vi "Stable.vi"(8 "Eval Period (sec)":dbl(knob)=0.5044674819294696 scale=0.0..1.0, 11 "Signal Input":bool) -> (0 "Stable":bool)   [LabVIEW 2011]
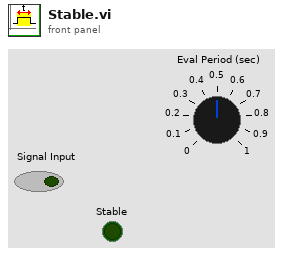
[diagram p1: front panel]
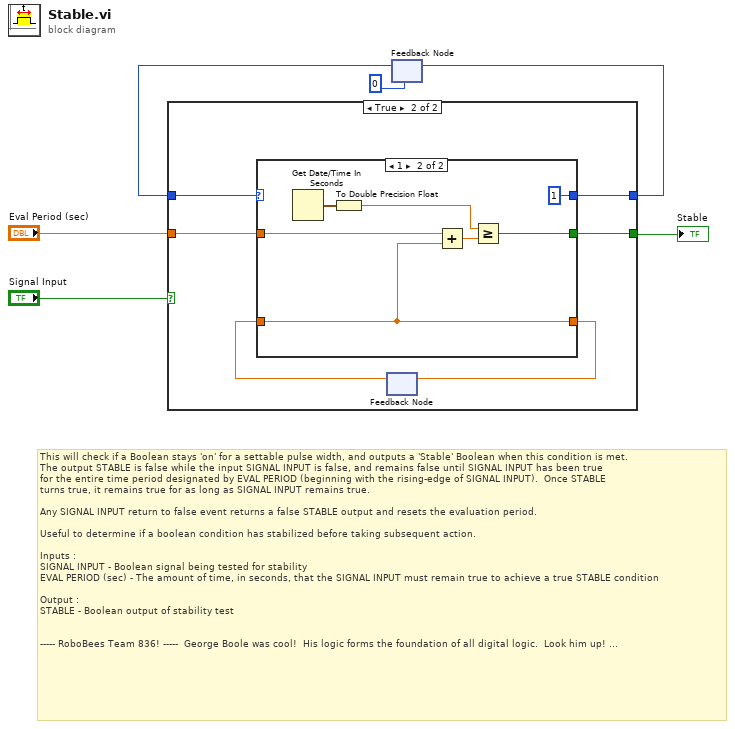
[diagram p0: block diagram]
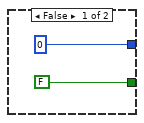
[diagram p2: hidden frame]
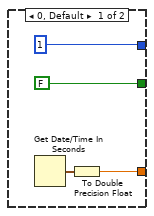
[diagram p3: hidden frame]
diagram:
  # "This will check if a Boolean stays 'on' for a settable pulse width, and outputs a 'Stable' Boolean when this condition is met.\nThe output STABLE is false while the input SIGNAL INPUT is false, and remains false until SIGNAL INPUT has been true\nfor the entire time period designated by EVAL PERIOD (beginning with the rising-edge of SIGNAL INPUT).  Once STABLE \nturns true, it remains true for as long as SIGNAL INPUT remains true.\n\nAny SIGNAL INPUT return to false event returns a false STABLE output and resets the evaluation period.\n\nUseful to determine if a boolean condition has stabilized before taking subsequent action.\n\nInputs :\nSIGNAL INPUT - Boolean signal being tested for stability\nEVAL PERIOD (sec) - The amount of time, in seconds, that the SIGNAL INPUT must remain true to achieve a true STABLE condition\n\nOutput :\nSTABLE - Boolean output of stability test\n\n\n----- RoboBees Team 836! -----  George Boole was cool!  His logic forms the foundation of all digital logic.  Look him up! ..."
  n1 = feedback #1(0) -> (w1:i32)
  n2 = case shown="True" "Signal Input" {
    tunnel: [FALSE w14] -> w6
    tunnel: "Eval Period (sec)" -> [_ w13]
    tunnel: [0 w10] -> w2
    tunnel: w1 -> [_ w9]
    frame False {
    }
    frame True {
      n3 = feedback #2() -> (w11:dbl)  [unwired: 1 in]
      n4 = case shown="1" w9 {
        tunnel: [FALSE w22] -> w14
        tunnel: w13 -> [_ w21]
        tunnel: [w16 w20] -> w12
        tunnel: w11 -> [_ w20]
        tunnel: [1 1] -> w10
        frame 0, Default {
          n5 = Get Date/Time In Seconds() -> (seconds since 1Jan1904=w17:timestamp)
          n6 = To Double Precision Float(number=w17) -> (double precision float=w16:dbl)
        }
        frame 1 {
          n7 = Get Date/Time In Seconds() -> (seconds since 1Jan1904=w25:timestamp)
          n8 = To Double Precision Float(number=w25) -> (double precision float=w23:dbl)
          n9 = Add(x=w21, y=w20) -> (x+y=w24:dbl)
          n10 = Greater Or Equal?(x=w23, y=w24) -> (x >= y?=w22:bool)
        }
      }
      n11 = feedback-in #2(w12) -> ()
    }
  }
  "Stable" <- w6
  n12 = feedback-in #1(w2) -> ()
